vi "Get Parameters File Needed Property.vi"(8 "error in":errorcluster, 11 "configuration files ref":T1 format="%.0x") -> (0 "error out":errorcluster, 2 "needed":bool, 3 "configuration files ref out":T1 format="%.0x")   [LabVIEW 2020, in "Ballard ARINC 429 Scripting.lvlib"]
uses:
  <vilib>/NI VeriStand/Custom Device API/Custom Device Item Ref.ctl
  Constants.vi
  Ballard ARINC 429 Scripting.lvlib
  <vilib>/NI VeriStand/Custom Device API/Custom Device API.lvlib
  <vilib>/NI VeriStand/Custom Device API/Get Item Property (Boolean).vi
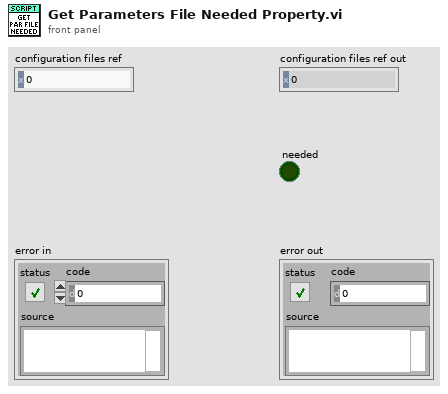
[diagram p1: front panel]
types:
  T1 = typedef "Custom Device API.lvlib/Custom Device Item Ref.ctl" = u64
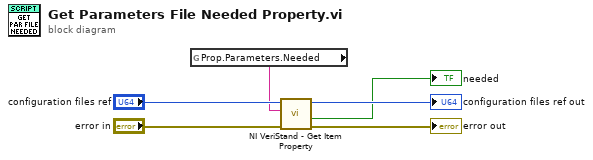
[diagram p0: block diagram]
diagram:
  n1 = global read "Constants.vi" "Prop.Parameters.Needed"() -> (w4:string)
  n2 = call-poly <vilib>:"NI VeriStand - Get Item Property.vi"("error in (no error)"="error in", "Property Name"=w4, "Item Ref in"="configuration files ref") -> ("error out"=→"error out":errorcluster, "Value"=→"needed":bool, "Item Ref out"=→"configuration files ref out":T1)  [unwired: 5 in, 1 out]
